vi "test_main.vi"() -> ()   [LabVIEW 2025]
uses:
  1cbc7890-2b9e-4b6b-a63a-61c39f236014.vi
panel:
  in  "Array":bool[](array[boolean])=[FALSE, FALSE, FALSE, FALSE, FALSE, FALSE, FALSE, FALSE, FALSE, FALSE, FALSE, FALSE, FALSE, FALSE, FALSE, FALSE, FALSE, FALSE, FALSE, FALSE, FALSE, FALSE, FALSE, FALSE, FALSE, FALSE, FALSE, FALSE, FALSE, FALSE, FALSE, FALSE, FALSE, FALSE, FALSE, FALSE, FALSE, FALSE, FALSE, FALSE, FALSE, FALSE, FALSE, FALSE, FALSE, FALSE, FALSE, FALSE, FALSE, FALSE, FALSE, FALSE, FALSE, FALSE, FALSE, FALSE, FALSE, FALSE, FALSE, FALSE, FALSE, FALSE, FALSE, FALSE, FALSE, FALSE, FALSE, FALSE, FALSE, FALSE, FALSE, FALSE, FALSE, FALSE, FALSE, FALSE, FALSE, FALSE, FALSE, FALSE, FALSE, FALSE, FALSE, FALSE, FALSE, FALSE, FALSE, FALSE, FALSE, FALSE, FALSE, FALSE, FALSE, FALSE, FALSE, FALSE, FALSE, FALSE, FALSE, FALSE]
  out "element":string
  out "keys":bool[](array[boolean])
  in  "stop":bool
  out "mode 2":u16
  in  "enter":bool
  in  "mode":u16(ring) items=["1 player", "AI vs. AI", "2 players (online)", "2 players (offline)"]
  in  "Reset":bool
  in  "Stop":bool
  out "screen":picture
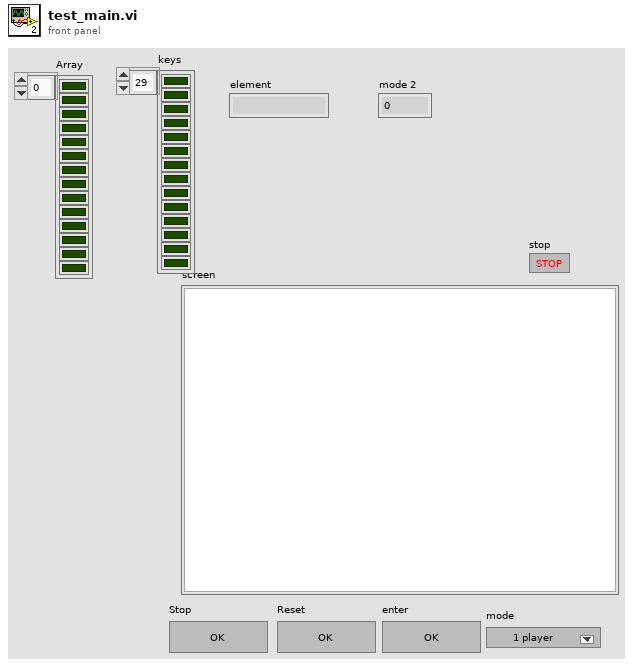
[diagram p1: front panel]
types:
  T1 = typedef "Sound Output Task ID.ctl" = u32
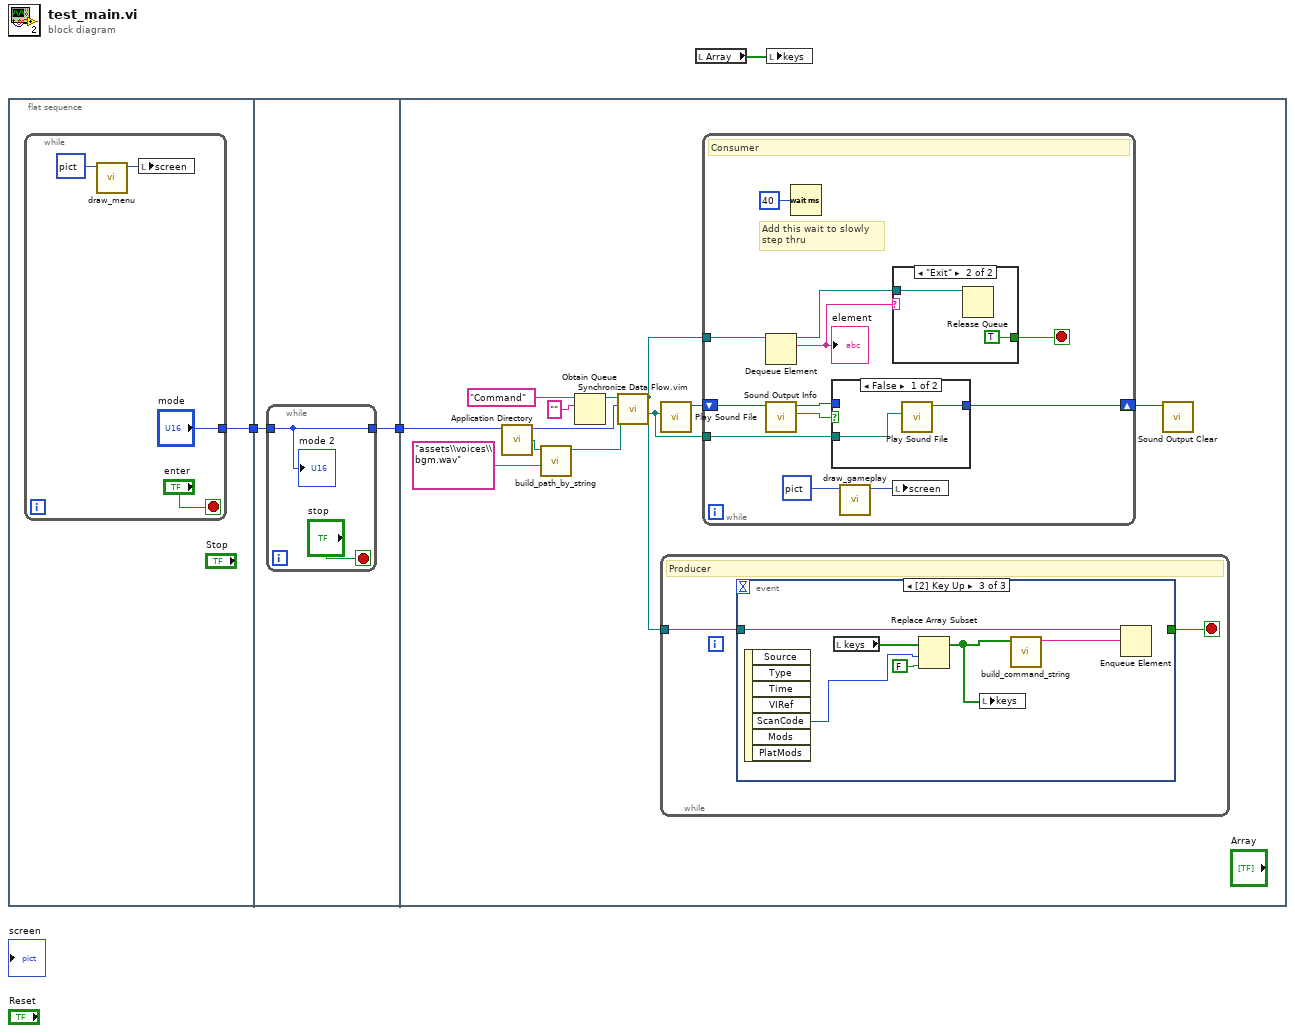
[diagram p0: block diagram]
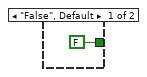
[diagram p3: hidden frame]
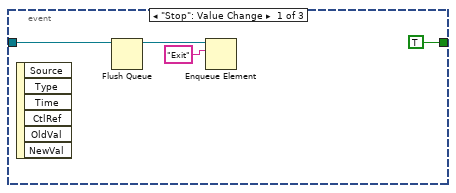
[diagram p4: hidden frame]
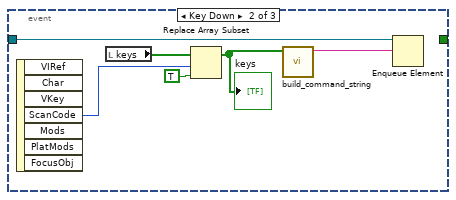
[diagram p5: hidden frame]
diagram:
  n1 = flat-sequence {
    tunnel: [w4] -> w3
    tunnel: w3 -> [w10]
    tunnel: [w9] -> w2
    tunnel: w2 -> [w16]
    frame #0 {
      n2 = while {
        tunnel: ["mode"] -> w4
        stop <- "enter" stop-if-true
        n3 = call "draw_menu.vi"("input"=picture data[5B]) -> ("menu"=w7:picture)  [unwired: 10 in]
        n4 = local write "screen"(w7) -> ()
      }
    }
    frame #1 {
      n5 = while {
        tunnel: w10 -> [w11]
        tunnel: [w11] -> w9
        stop <- "stop" stop-if-true
        "mode 2" <- w11
      }
    }
    frame #2 {
      n6 = call <vilib>:"Application Directory.vi"() -> ("Application Directory"=w17:path)
      n7 = call "build_path_by_string.vi"("String"="assets\\voices\\bgm.wav", "base path"=w17) -> ("appended path"=w22:path)  [unwired: 9 in]
      n8 = Obtain Queue(name (unnamed)="Command", element data type="" ("name (unnamed)")) -> (queue out=w20:refnum<queue>)  [unwired: 3 in, 2 out]
      n9 = call "Synchronize Data Flow.vim"("input 3"=w22, "input 2"=w16, "input 1"=w20) -> ("output 3"=w23:path, "output 1"=w21:refnum<queue>)  [unwired: 1 in, 2 out]
      n10 = call <vilib>:"Play Sound File.vi"("path"=w23) -> ("task ID"=w18:T1)  [unwired: 9 in, 1 out]
      n11 = while {
        tunnel: w21 -> [w42]
        stop <- w43 stop-if-true
        # "Producer"
        n12 = event shown="[2] Key Up" {
          selector: _ -> [_ _ _]
          dyn-events: _ -> [_ _ _]
          timeout: _ -> [_ _ _]
          tunnel: [TRUE _ _] -> w43
          tunnel: w42 -> [w45 w50 w57]
          event "Stop": Value Change {
            n13 = event-data() -> ()  [unwired: 1 in, 6 out]
            n14 = Flush Queue(queue=w45) -> (queue out=w44:refnum<queue>)  [unwired: 1 in, 2 out]
            n15 = Enqueue Element(queue=w44, element="Exit") -> ()  [unwired: 2 in, 3 out]
          }
          event Key Down {
            n16 = event-data() -> ("ScanCode"=w52:i16)  [unwired: 1 in, 6 out]
            n17 = local read "keys"() -> (w53:bool[])
            n18 = Replace Array Subset(array=w53, new element=TRUE ("new element/subarray"), index=w52) -> (w49:bool[])
            "keys" <- w49
            n19 = call "build_command_string.vi"("key state"=w49) -> ("command"=w48:string)  [unwired: 10 in]
            n20 = Enqueue Element(queue=w50, element=w48) -> ()  [unwired: 2 in, 3 out]
          }
          event Key Up {
            n21 = event-data() -> ("ScanCode"=w56:i16)  [unwired: 1 in, 6 out]
            n22 = local read "keys"() -> (w59:bool[])
            n23 = Replace Array Subset(array=w59, new element=FALSE ("new element/subarray"), index=w56) -> (w54:bool[])
            n24 = local write "keys"(w54) -> ()
            n25 = call "build_command_string.vi"("key state"=w54) -> ("command"=w55:string)  [unwired: 10 in]
            n26 = Enqueue Element(queue=w57, element=w55) -> ()  [unwired: 2 in, 3 out]
          }
        }
      }
      n27 = while {
        tunnel: w21 -> [w35]
        shift-right: [w28] -> w19
        shift-left: w18 -> [w27]
        tunnel: w23 -> [w26]
        stop <- w32 stop-if-true
        # "Add this wait to slowly step thru"
        # "Consumer"
        n28 = Dequeue Element(queue=w35) -> (queue out=w33:refnum<queue>, element=w31:string)  [unwired: 2 in, 2 out]
        "element" <- w31
        n29 = call <vilib>:"Sound Output Info.vi"("task ID"=w27) -> ("is playing?"=w30:bool, "task ID out"=w29:T1)  [unwired: 7 in, 2 out]
        n30 = Wait (ms)(milliseconds to wait=u32 40) -> ()  [unwired: 1 out]
        n31 = case shown="False" w30 {
          tunnel: w26 -> [w37 _]
          tunnel: [w36 w38] -> w28
          tunnel: w29 -> [_ w38]
          frame False {
            n32 = call <vilib>:"Play Sound File.vi"("path"=w37) -> ("task ID"=w36:T1)  [unwired: 9 in, 1 out]
          }
          frame True {
          }
        }
        n33 = call "draw_gameplay.vi"("input"=picture data[5B]) -> ("gameplay"=w25:picture)  [unwired: 10 in]
        n34 = case shown="\"Exit\"" w31 {
          tunnel: w33 -> [_ w41]
          tunnel: [FALSE TRUE] -> w32
          frame "False", Default {
          }
          frame "Exit" {
            n35 = Release Queue(queue=w41) -> ()  [unwired: 2 in, 3 out]
          }
        }
        n36 = local write "screen"(w25) -> ()
      }
      n37 = call <vilib>:"Sound Output Clear.vi"("task ID"=w19) -> ()  [unwired: 10 in, 1 out]
    }
  }
  n38 = local read "Array"() -> (w1:bool[])
  n39 = local write "keys"(w1) -> ()
